vi "Read Error Queue.vi"(7 "FIFO Debug Flags":refnum<class "FIFO Flags.lvclass">, 8 "error in (no error)":errorcluster, 9 "timeout in ms (0)":i32 format="%d ms", 11 "Error Queue in":T1) -> (0 "error out":errorcluster, 1 "timed out?":bool, 2 "element":errorcluster, 3 "Error Queue out":T1)   [LabVIEW 2017, in "DSF Core.lvlib" / "Interface.lvclass"]
uses:
  Interface.lvclass
  Error Queue Ref.ctl
  Debug/FIFO Flags/FIFO Flags.lvclass
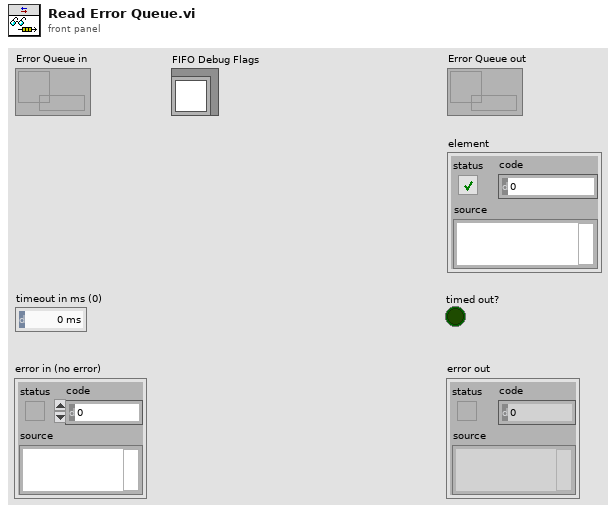
[diagram p1: front panel]
types:
  T1 = typedef "DSF Core.lvlib/Interface.lvclass/Error Queue Ref.ctl" = refnum<queue>
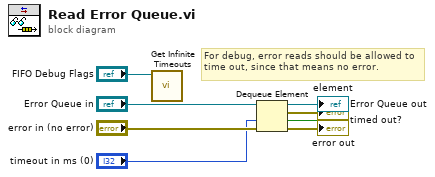
[diagram p0: block diagram]
diagram:
  # "For debug, error reads should be allowed to time out, since that means no error."
  n1 = call "Get Infinite Timeouts.vi"("FIFO Debug Flags in"="FIFO Debug Flags") -> ()  [unwired: 9 in, 2 out]
  n2 = Dequeue Element(queue="Error Queue in", timeout in ms (-1)="timeout in ms (0)", error in (no error)="error in (no error)") -> (queue out=→"Error Queue out":T1, element=→"element":errorcluster, timed out?=→"timed out?":bool, error out=→"error out":errorcluster)
